vi "InvalidRefError.vi"(8 "error in (no error)":errorcluster, 11 "VI Name":string) -> (0 "error out":errorcluster)   [LabVIEW 2017, in "Watchdog.lvclass"]
uses:
  <vilib>/NI/Software Watchdog/Watchdog/Watchdog.lvclass
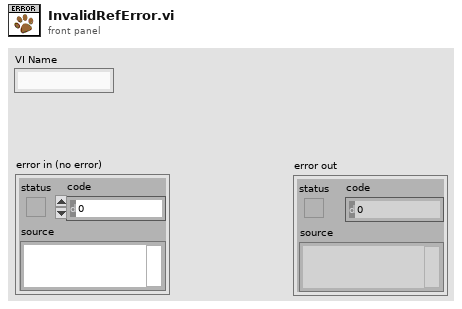
[diagram p1: front panel]
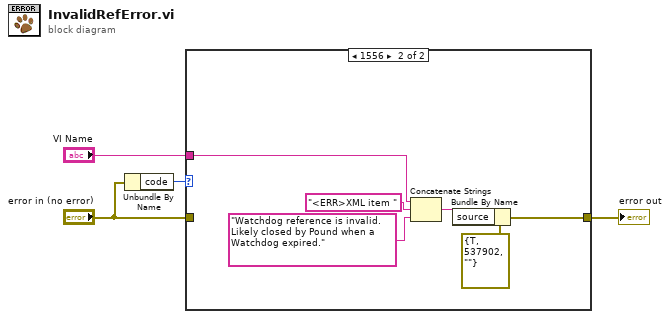
[diagram p0: block diagram]
diagram:
  n1 = Unbundle By Name("error in (no error)") -> ("code"=w3:i32)
  n2 = case shown="1556" w3 {
    tunnel: [w5 w7] -> w4
    tunnel: "error in (no error)" -> [w5 _]
    tunnel: "VI Name" -> [_ w6]
    frame 0, Default {
    }
    frame 1556 {
      n3 = Concatenate Strings(w6, "<ERR>XML item " ("Format String"), "Watchdog reference is invalid.  Likely closed by Pound when a Watchdog expired.") -> (w10:string)
      n4 = Bundle By Name(cluster=errorcluster {"status"=TRUE, "code"=537902, "source"=""} ("error in"), "source"=w10) -> (w7:errorcluster)
    }
  }
  "error out" <- w4
